vi "Excel Write Profile.vi"(8 "Error In":errorcluster, 9 "CMD Step":dbl format="%#_13g", 10 "Profile":string[][](array[string]), 11 "Cells Ref In":refnum<k7>) -> (0 "Error Out":errorcluster, 3 "Cells Ref Out":refnum<k7>)   [LabVIEW 2013]
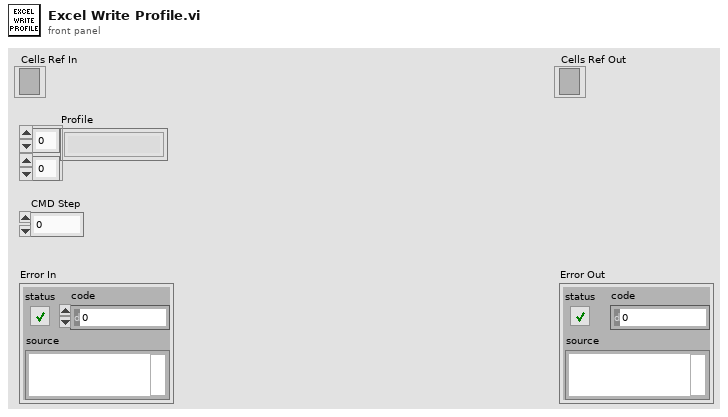
[diagram p1: front panel]
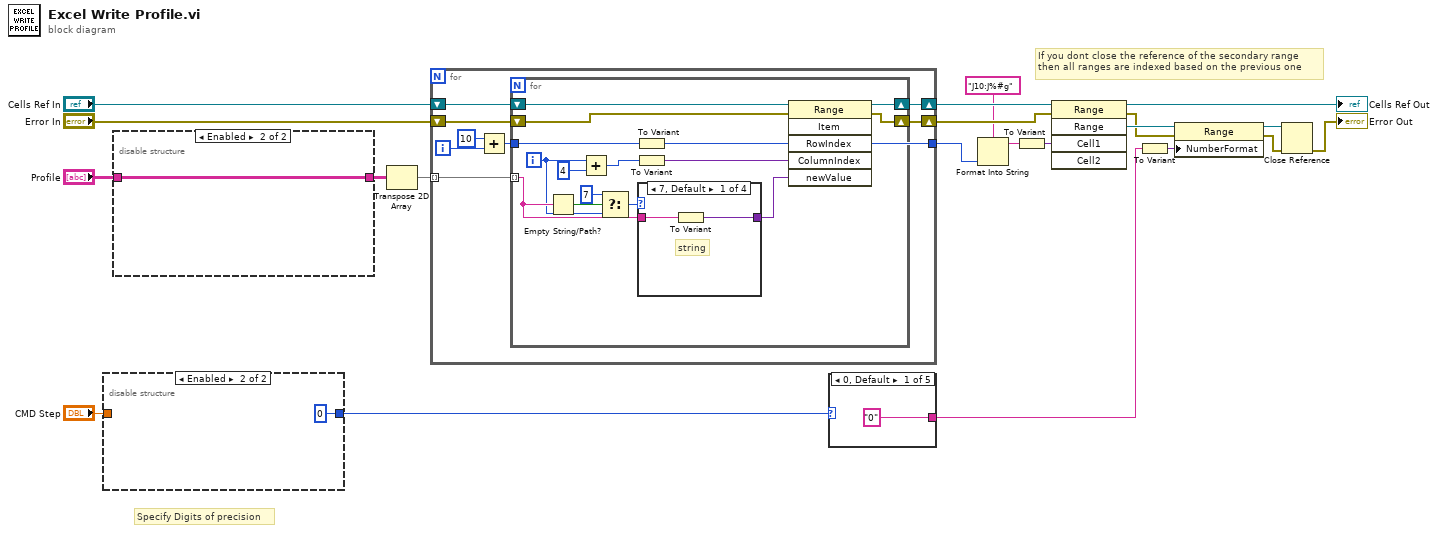
[diagram p0: block diagram]
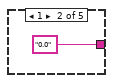
[diagram p3: hidden frame]
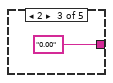
[diagram p4: hidden frame]
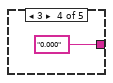
[diagram p5: hidden frame]
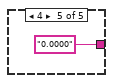
[diagram p6: hidden frame]
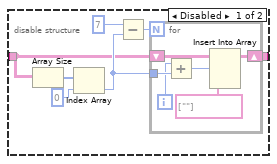
[diagram p7: hidden frame]
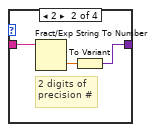
[diagram p8: hidden frame]
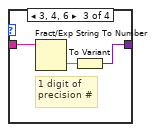
[diagram p9: hidden frame]
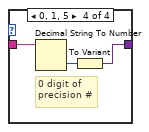
[diagram p10: hidden frame]
diagram:
  # "Specify Digits of precision"
  # "If you dont close the reference of the secondary range\nthen all ranges are indexed based on the previous one"
  n1 = disable-structure shown="Enabled" {
    disable-tunnel: [_ 0 ("Digits of Significance")] -> w16
    disable-tunnel: "CMD Step" -> [_ _]
    frame Disabled {
    }
    frame Enabled {
    }
  }
  n2 = disable-structure shown="Enabled" {
    disable-tunnel: [w29 w36] -> w19
    disable-tunnel: "Profile" -> [w23 w36]
    frame Disabled {
      n3 = Array Size(array=w23) -> (size(s)=w24:i32[])
      n4 = Index Array(array=w24, index=0) -> (element=w28:i32)
      n5 = Subtract(x=7 ("y"), y=w28) -> (x-y=w27:i32)
      n6 = for {
        N: w27 -> [_]
        shift-right: [w33] -> w29
        shift-left: w23 -> [w34]
        tunnel: w28 -> [w31]
        i -> [w30]
        n7 = Add(x=w30, y=w31) -> (x+y=w32:i32)
        n8 = Insert Into Array(array=w34, index (row)=w32, new element=string[] [""]) -> (w33:string[][])  [unwired: 1 in]
      }
    }
    frame Enabled {
    }
  }
  n9 = Transpose 2D Array(2D array=w19) -> (transposed array=w18:string[][])
  n10 = for {
    shift-right: [w42] -> w7
    shift-left: "Cells Ref In" -> [w41]
    shift-right: [w43] -> w5
    shift-left: "Error In" -> [w40]
    tunnel: w18 -> [w44] mode=indexing
    tunnel: [w37] -> w1
    i -> [w38]
    n11 = Add(x=10, y=w38) -> (x+y=w37:i32)
    n12 = for {
      shift-right: [w58] -> w42
      shift-left: w41 -> [w59]
      shift-right: [w57] -> w43
      shift-left: w40 -> [w56]
      tunnel: w44 -> [w52] mode=indexing
      tunnel: w37 -> [w45]
      i -> [w48]
      n13 = Empty String/Path?(string/path=w52) -> (empty?=w51:bool)
      n14 = Add(x=w48, y=4) -> (x+y=w47:i32)
      n15 = Select(t=7, s=w51, f=w48) -> (s? t:f=w49:i32)
      n16 = To Variant(anything=w45) -> (Variant=w55:variant)
      n17 = To Variant(anything=w47) -> (Variant=w54:variant)
      n18 = case shown="7, Default" w49 {
        tunnel: w52 -> [w61 w64 w67 w70]
        tunnel: [w60 w62 w65 w68] -> w53
        frame 7, Default {
          # "string"
          n19 = To Variant(anything=w61) -> (Variant=w60:variant)
        }
        frame 2 {
          # "2 digits of\nprecision #"
          n20 = Fract/Exp String To Number(string=w64) -> (number=w63:dbl)  [unwired: 3 in, 1 out]
          n21 = To Variant(anything=w63) -> (Variant=w62:variant)
        }
        frame 3, 4, 6 {
          # "1 digit of\nprecision #"
          n22 = Fract/Exp String To Number(string=w67) -> (number=w66:dbl)  [unwired: 3 in, 1 out]
          n23 = To Variant(anything=w66) -> (Variant=w65:variant)
        }
        frame 0, 1, 5 {
          # "0 digit of\nprecision #"
          n24 = Decimal String To Number(string=w70) -> (number=w69:i32)  [unwired: 2 in, 1 out]
          n25 = To Variant(anything=w69) -> (Variant=w68:variant)
        }
      }
      n26 = invoke class="Range" method="Item"(reference=w59, error in=w56, "RowIndex"=w55, "ColumnIndex"=w54, "newValue"=w53) -> (reference out=w58:refnum<k7>, error out=w57:errorcluster)  [unwired: 1 in, 4 out]
    }
  }
  n27 = case shown="0, Default" w16 {
    tunnel: ["0" "0.0" "0.00" "0.000" "0.0000"] -> w2
    frame 0, Default {
    }
    frame 1 {
    }
    frame 2 {
    }
    frame 3 {
    }
    frame 4 {
    }
  }
  n28 = Format Into String(format string="J10:J%#g", w1) -> (resulting string=w14:string)  [unwired: 2 in, 1 out]
  n29 = To Variant(anything=w14) -> (Variant=w12:variant)
  n30 = invoke class="Range" method="Range"(reference=w7, error in=w5, "Cell1"=w12) -> (reference out=→"Cells Ref Out":refnum<k7>, error out=w10:errorcluster, "Range"=w11:refnum<k7>)  [unwired: 2 in, 2 out]
  n31 = To Variant(anything=w2) -> (Variant=w13:variant)
  n32 = property class="Range"(reference=w11, error in=w10, "NumberFormat"=w13) -> (reference out=w9:refnum<k7>, error out=w8:errorcluster)
  n33 = Close Reference(reference=w9, error in (no error)=w8) -> (error out=→"Error Out":errorcluster)
